vi "alignAudioVideoQueues.vi"(7 "Image pointer recycling queue":refnum<queue>, 8 "error in (no error)":errorcluster, 9 "Alignment tolerance":dbl, 10 "Video queue in":refnum<queue>, 11 "Audio queue in":refnum<queue>) -> (0 "error out":errorcluster, 2 "Video queue out":refnum<queue>, 3 "Audio queue out":refnum<queue>, 5 "Image pointer recycling queue out":refnum<queue>)   [LabVIEW 2017]
uses:
  <vilib>/vision/Image Controls.llb/IMAQ Image.ctl
panel:
  out "Video timestamps":timestamp[](array[timestamp]) format="%<%I:%M:%S%3u %p>T"
  out "Audio timestamps":timestamp[](array[timestamp]) format="%<%I:%M:%S%3u %p>T"
  out "Video frames shed":i32
  out "Audio chunks shed":i32
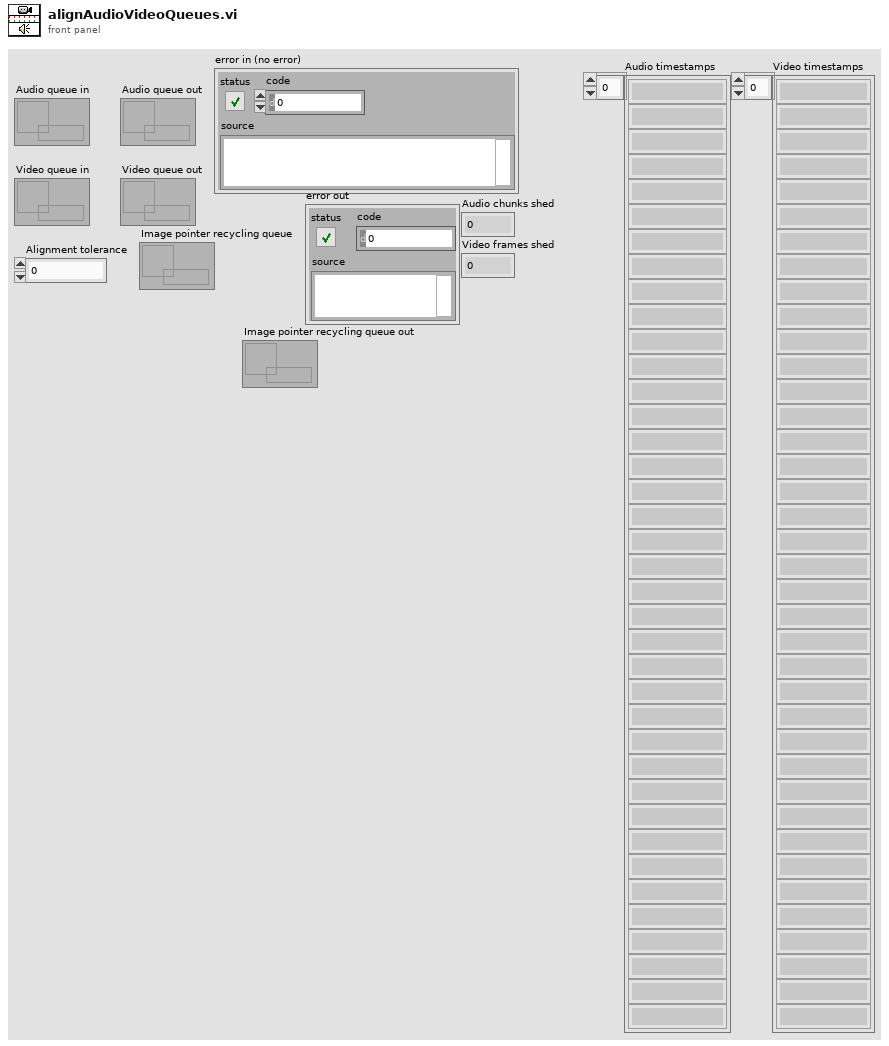
[diagram p1: front panel]
types:
  T1 = typedef "IMAQ Image.ctl" = refnum<image>
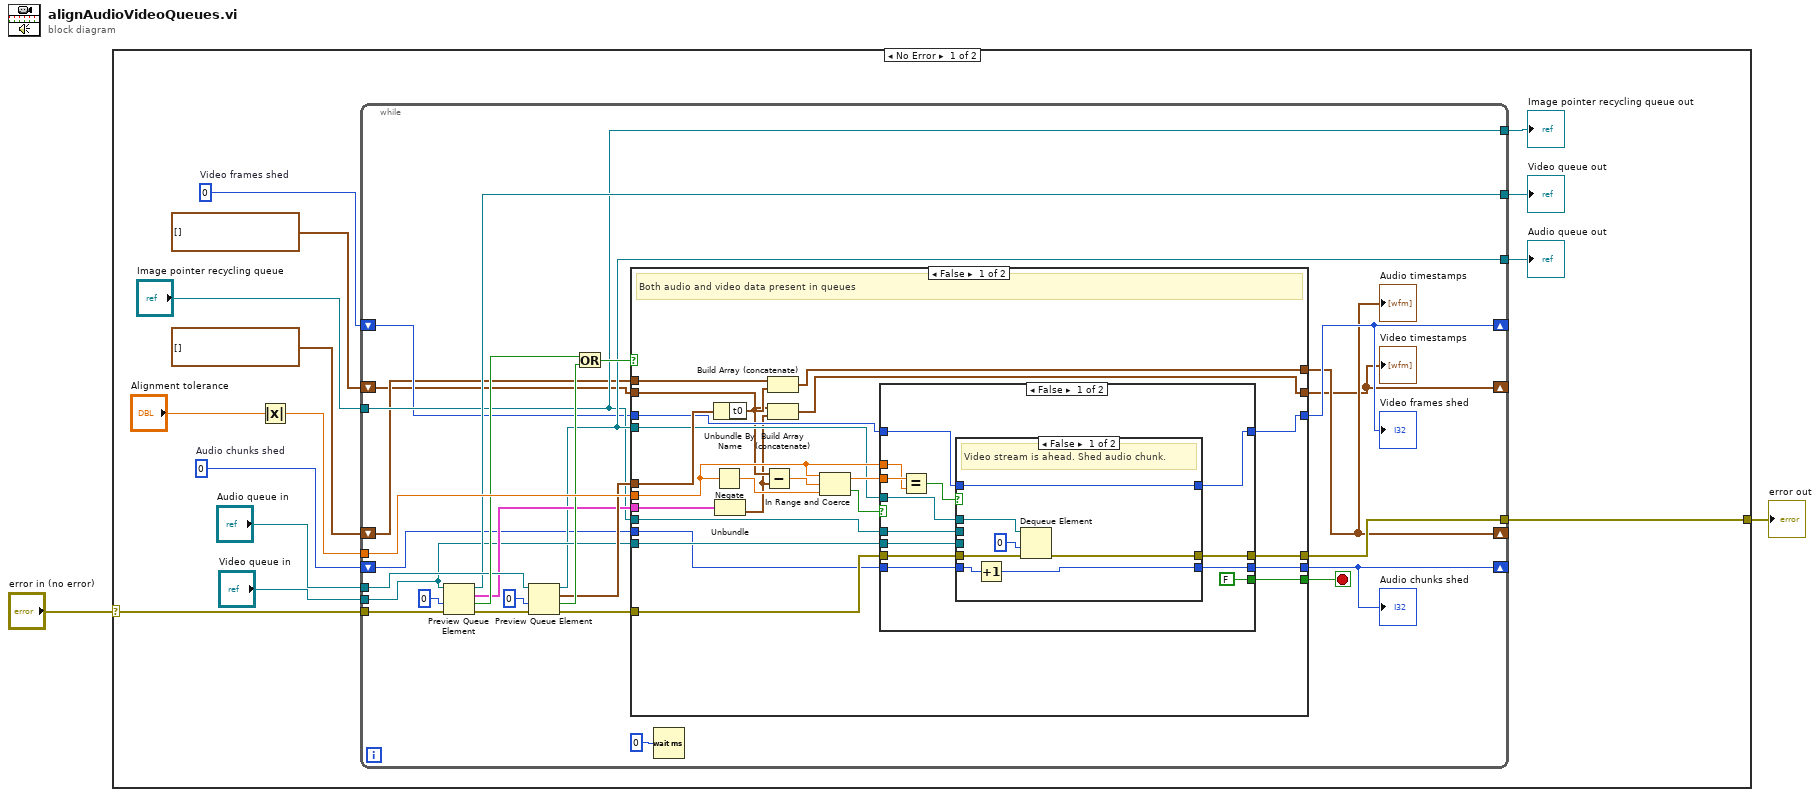
[diagram p0: block diagram]
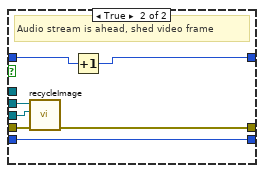
[diagram p2: hidden frame]
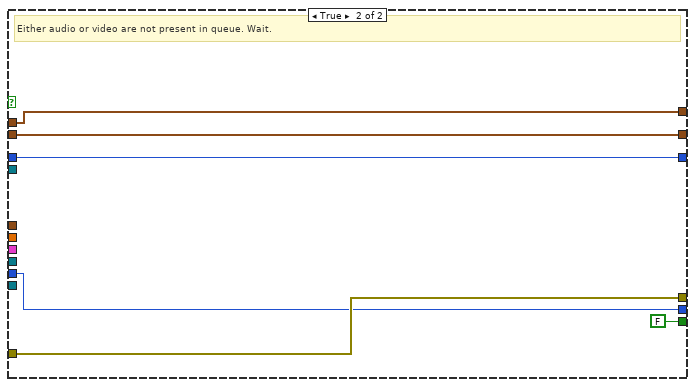
[diagram p4: hidden frame]
diagram:
  n1 = case shown="No Error" "error in (no error)" {
    selector: "error in (no error)" -> [w9 w104]
    tunnel: [w8 w104] -> w1
    frame No Error {
      w6 = 0  # Audio chunks shed
      w5 = 0  # Video frames shed
      n2 = Absolute Value(x="Alignment tolerance") -> (abs(x)=w10:dbl)
      n3 = while {
        tunnel: w10 -> [w43]
        tunnel: "Audio queue in" -> [w38]
        tunnel: "Video queue in" -> [w32]
        tunnel: [w33] -> w13
        tunnel: [w31] -> w12
        tunnel: "Image pointer recycling queue" -> [w25]
        tunnel: w9 -> [w28]
        tunnel: [w30] -> w8
        tunnel: [w25] -> w7
        shift-right: [w22] -> _
        shift-left: w5 -> [w24]
        shift-right: [w21] -> _
        shift-left: w6 -> [w23]
        shift-right: [w18] -> _
        shift-left: timestamp[] [] -> [w20]
        shift-right: [w17] -> _
        shift-left: timestamp[] [] -> [w19]
        stop <- w34 stop-if-true
        n4 = Preview Queue Element(queue=w32, timeout in ms (-1)=0, error in (no error)=w28) -> (queue out=w33:refnum<queue>, element=w36:cluster{"Image Out":T1, timestamp}, timed out?=w40:bool, error out=w29:errorcluster)
        n5 = Preview Queue Element(queue=w38, timeout in ms (-1)=0, error in (no error)=w29) -> (queue out=w31:refnum<queue>, element=w39:waveform(dbl), timed out?=w41:bool, error out=w27:errorcluster)
        n6 = Or(x=w40, y=w41) -> (x .or. y?=w42:bool)
        n7 = case shown="False" w42 {
          tunnel: w36 -> [w66 _]
          tunnel: w39 -> [w65 _]
          tunnel: w43 -> [w59 _]
          tunnel: [w61 FALSE] -> w34
          tunnel: w25 -> [w58 _]
          tunnel: w32 -> [w57 _]
          tunnel: w31 -> [w56 _]
          tunnel: w27 -> [w55 w102]
          tunnel: [w54 w102] -> w30
          tunnel: w24 -> [w53 w100]
          tunnel: w23 -> [w52 w101]
          tunnel: [w51 w100] -> w22
          tunnel: [w50 w101] -> w21
          tunnel: w20 -> [w49 w99]
          tunnel: w19 -> [w47 w98]
          tunnel: [w45 w99] -> w18
          tunnel: [w44 w98] -> w17
          frame False {
            # "Both audio and video data present in queues"
            n8 = Unbundle By Name(w65) -> ("t0"=w48:timestamp)
            n9 = Negate(x=w59) -> (-x=w63:dbl)
            n10 = Unbundle(w66) -> (w46:timestamp)  [unwired: 1 out]
            n11 = Subtract(x=w48, y=w46) -> (x-y=w64:dbl)
            n12 = Build Array (concatenate)(w49, w48) -> (w45:timestamp[])
            n13 = Build Array (concatenate)(w47, w46) -> (w44:timestamp[])
            n14 = In Range and Coerce(upper limit=w59, x=w64, lower limit=w63) -> (coerced(x)=w60:dbl, In Range?=w62:bool)
            n15 = case shown="False" w62 {
              selector: w62 -> [_ w97]
              tunnel: [FALSE w97] -> w61
              tunnel: w60 -> [w78 _]
              tunnel: w59 -> [w77 _]
              tunnel: w58 -> [w75 _]
              tunnel: w57 -> [w74 _]
              tunnel: w56 -> [w73 _]
              tunnel: w55 -> [w72 w96]
              tunnel: [w71 w96] -> w54
              tunnel: w53 -> [w70 w94]
              tunnel: w52 -> [w69 w95]
              tunnel: [w68 w94] -> w51
              tunnel: [w67 w95] -> w50
              frame False {
                n16 = Equal?(x=w78, y=w77) -> (x = y?=w76:bool)
                n17 = case shown="False" w76 {
                  tunnel: w75 -> [_ w93]
                  tunnel: w74 -> [_ w92]
                  tunnel: w73 -> [w86 _]
                  tunnel: w72 -> [w84 w90]
                  tunnel: [w83 w91] -> w71
                  tunnel: w70 -> [w80 w89]
                  tunnel: w69 -> [w82 w87]
                  tunnel: [w80 w88] -> w68
                  tunnel: [w81 w87] -> w67
                  frame False {
                    # "Video stream is ahead. Shed audio chunk."
                    n18 = Increment(x=w82) -> (x+1=w81:i32)
                    n19 = Dequeue Element(queue=w86, timeout in ms (-1)=0, error in (no error)=w84) -> (error out=w83:errorcluster)  [unwired: 3 out]
                  }
                  frame True {
                    # "Audio stream is ahead, shed video frame"
                    n20 = call "recycleImage.vi"("error in (no error)"=w90, "Video queue"=w92, "Image pointer recylcing queue"=w93) -> ("error out"=w91:errorcluster)  [unwired: 8 in]
                    n21 = Increment(x=w89) -> (x+1=w88:i32)
                  }
                }
              }
              frame True {
                # "Queues are aligned"
              }
            }
          }
          frame True {
            # "Either audio or video are not present in queue. Wait."
          }
        }
        "Audio chunks shed" <- w21
        "Video frames shed" <- w22
        "Audio timestamps" <- w18
        "Video timestamps" <- w17
        n22 = Wait (ms)(milliseconds to wait=u32 0) -> ()  [unwired: 1 out]
      }
      "Audio queue out" <- w12
      "Video queue out" <- w13
      "Image pointer recycling queue out" <- w7
    }
    frame Error {
    }
  }
  "error out" <- w1
